vi "Read Element of Channel Names.vi"(8 "error in (no error)":errorcluster, 10 "index":i32, 11 "Lakeshore 325 in":refnum<class "Lakeshore 325.lvclass">) -> (0 "error out":errorcluster, 2 "?":string, 3 "Lakeshore 325 out":refnum<class "Lakeshore 325.lvclass">)   [LabVIEW 2022 SP3, in "Lakeshore 325.lvclass"]
uses:
  Lakeshore 325.lvclass
  Lakeshore 325.lvclass/Lakeshore 325.ctl
  Temp Control.lvclass
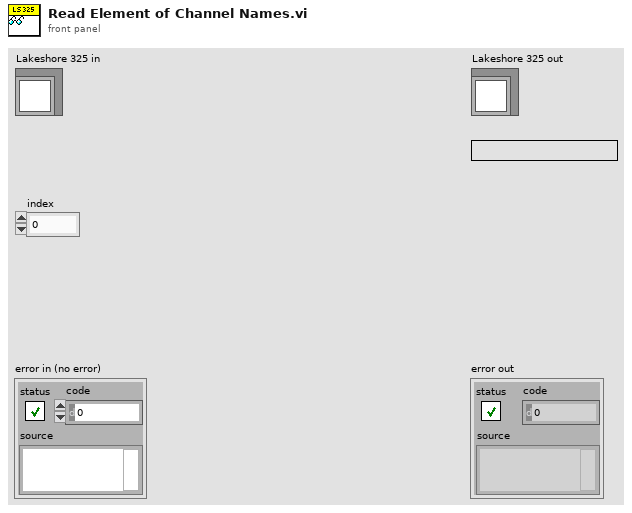
[diagram p1: front panel]
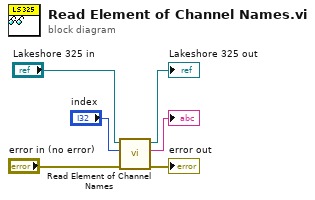
[diagram p0: block diagram]
diagram:
  n1 = call-parent "Read Element of Channel Names.vi"("error in (no error)"="error in (no error)", "index"="index", "Temp Control in"="Lakeshore 325 in") -> ("error out"=→"error out":errorcluster, 2:→"?":string, "Temp Control out"=→"Lakeshore 325 out":refnum<class "Lakeshore 325.lvclass">)  [unwired: 6 in]
